vi "多进制显示数值控件.vi"() -> ()   [LabVIEW 2012]
panel:
  out "数值显示控件":i32 format="  2进制：%b\n10进制：%d\n16进制:  %x"
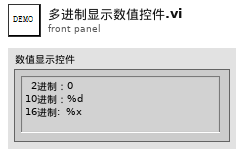
[diagram p1: front panel]
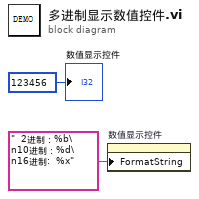
[diagram p0: block diagram]
diagram:
  n1 = property on="数值显示控件" class="DigNum (严格)"("FormatString"="  2进制：%b\n10进制：%d\n16进制:  %x" ("格式字符串")) -> ()  [unwired: 2 in, 2 out]
  "数值显示控件" <- 123456 ("数值显示控件")
